vi "MultiplexDAQ_Main.vi"() -> ()   [LabVIEW 2011]
uses:
  controls/General Hardware config.ctl
  controls/DAQ Setup.ctl
  controls/PlotProperties.ctl
  controls/SampleClockExport.ctl
  controls/AnalogOutputSetup.ctl
  controls/RefClockSettings.ctl
  controls/Counter Setup.ctl
  controls/ProgramStatus.ctl
  <vilib>/Utility/miscctls.llb/LVBoundsTypeDef.ctl
  <vilib>/Utility/miscctls.llb/LVPointTypeDef.ctl
  <vilib>/Utility/miscctls.llb/LVRectTypeDef.ctl
  controls/XmlOption.ctl
  <vilib>/DAQmx/write.llb/DAQmx Write (Analog 1D DBL NChan 1Samp).vi
  <vilib>/DAQmx/read.llb/DAQmx Read (Analog 2D DBL NChan NSamp).vi
  <vilib>/DAQmx/miscellaneous.llb/DAQmx Fill In Error Info.vi
  C:/Program Files/National Instruments/LabVIEW 2011/resource/objmgr/daqmx.rc
panel:
  out "XMLConfigControls":refnum<vi>[](array[refnum])
  out "DisableDuringRecord":refnum<vi>[](array[refnum])
  in  "TDMS Group Name":string="MultiplexRecord"
  out "BufferStatus":u32[](array[colorbox])
  out "DisableDuringRun":refnum<vi>[](array[refnum])
  out "AllTasks":T1
  out "KillEvent":refnum<user-event>[](array[refnum])
  in  "Tab Control":T2(tab)=enum."Raw Signal"
  in  "Note":string
  out "Recording Time":string
  out "Index":i32
  in  "Menu Ring":enum16{"Manual", "Column"}(ring)
  in  "Up Button":bool
  in  "Down Button":bool
  in  "Preview?":bool
  in  "OverWrite?":bool
  in  "StartRecord":bool
  out "Amplitude Scale":dbl
  out "Effective Sampling Rate":dbl
  in  "Plot Properties":T3={"First Index"=0, "Last Index"=10, "Time (sec)"=1.0, "Zoom Factor"=1.0, "SubtractMean?"=FALSE, "DisplayOption"=enum."Scroll"} {"Zoom Factor" min=0.0 max=1.0}
  in  "TDMS file path":path=path "C:/Users/DAQ/Desktop/test_001.tdms"
  out "Waveform Graph":dbl[][](graph)
  in  "AutoNr":bool
  in  "SingleRaw?":bool
  in  "AC/DC Select":T4(ring)
  in  "WindowSize":i32=1 caption="(s)  Window Size For Averaging" min=1 max=10
  out "Intensity Graph":dbl[][](graph) caption="Array"
  in  "Row/Col Index":dbl caption="Select the Row/Col Index" min=0.0
  in  "Row/Col Select":enum16{"Show single column", "Show single row"}(ring)
  out "DC Offset":dbl[](graph) caption="Mean of Signal during window"
  out "AC_Range":dbl[](graph) caption="Standard Deviation of Signal during window"
  out "Raw Signal":dbl[](graph)
  in  "Raw Channel":i32=6 caption="Select Column" min=0
  in  "Open Button":bool
  in  "Save Button":bool
  in  "LUT":i32[](array[numeric]) caption="Channel Mix Vector"
  in  "BitSwitch":bool=TRUE caption="Switch most/least Significant bit"
  in  "HWSettings":T5={"Nr. of Columns"=1, "Nr. of Rows"=18, "OverSampling"=10, "Fetch Rate "=20, "Sampling Rate"=50000, "Nr. of BNC inputs"=3, "Sample Strip Length"=1} caption="Hardware Settingss"
  out "Smpls per Poll":i32 caption="Effective samples \nper poll"
  out "Smpls per CH*poll":i32 caption="Smpls per channel \nper poll"
  in  "AnalogSettings":T6=[{"AnalogOut (Volt)"=[5.0, 5.0, 5.0, 5.0], "DAQmx Device Name"="PXI1Slot2"}, {"AnalogOut (Volt)"=[5.0, 5.0, 5.0, 5.0], "DAQmx Device Name"="PXI1Slot3"}, {"AnalogOut (Volt)"=[5.0, 5.0, 5.0, 5.0], "DAQmx Device Name"="PXI1Slot6"}] caption="Analog Output Voltage Setup"
  in  "Digital Out Tasks":tag[](array[tag])=["PXI1Slot2/port0", "PXI1Slot3/port0", "PXI1Slot6/port0"]
  in  "Referece Clock Setup":T7={"RefClockGlobalName"="PXI_Clk10", "RefClockRate"=10000000.0}
  in  "Counter Setup":T8={"Device and Counter"="PXI1Slot3/ctr0", "PXI_trigger"="PXI_Trig3"}
  in  "RowConfigFile":path=path "C:/Users/DAQ/Desktop/Labview Joost/MultiplexDAQ/ConfigFiles/DecBinVals_L2R.txt" caption="Row Select Configuration file"
  in  "AnalogInSettings":T9[](array[typedef])=[{"Input Voltage Range"=10.0, "Upsample Coefficient"=1, "Analog Input Channels"="PXI1Slot2/ai0:7", "Configuration"=10106}, {"Input Voltage Range"=10.0, "Upsample Coefficient"=1, "Analog Input Channels"="PXI1Slot3/ai0:7", "Configuration"=10106}, {"Input Voltage Range"=10.0, "Upsample Coefficient"=2, "Analog Input Channels"="PXI1Slot6/ai0:4", "Configuration"=10106}] caption="Analog Input Tasks per PXI device" {"Configuration" items=["Differential"=10106, "RSE"=10083, "NRSE"=10078, "Pseudodifferential"=12529]}
  out "Digital Out BitMask":bool[][][](array[boolean])
  in  "Sample Clock Export":T10={"DAQmx Terminal"="/PXI1Slot2/PFI0", "ExportClock?"=FALSE, "DAQmx Device Name"="PXI1Slot2"}
  # "Plot Window Settings"
  # "V/unit"
  # "Hz"
  # "Disclaimer:\nThe mean and standard deviation\nthat are displayed in the graphs are\nan approximation of the real mean\nand standard deviation. \n\nUse Matlab to calculate the real values\nif they are important."
  # "Analog Input Settings"
  # "Analog Output Settings"
  # "General Hardware Settings"
  # "Row Select Digital Output Setting"
  # "Array"
  # "Acq. System"
  # "Other analog Input"
  # "You can export the sampling clock of any task to a DAQmx terminal. This is usefull for testing with the scope."
  # "Select PXI card"
  # "Time"
  # "Bit"
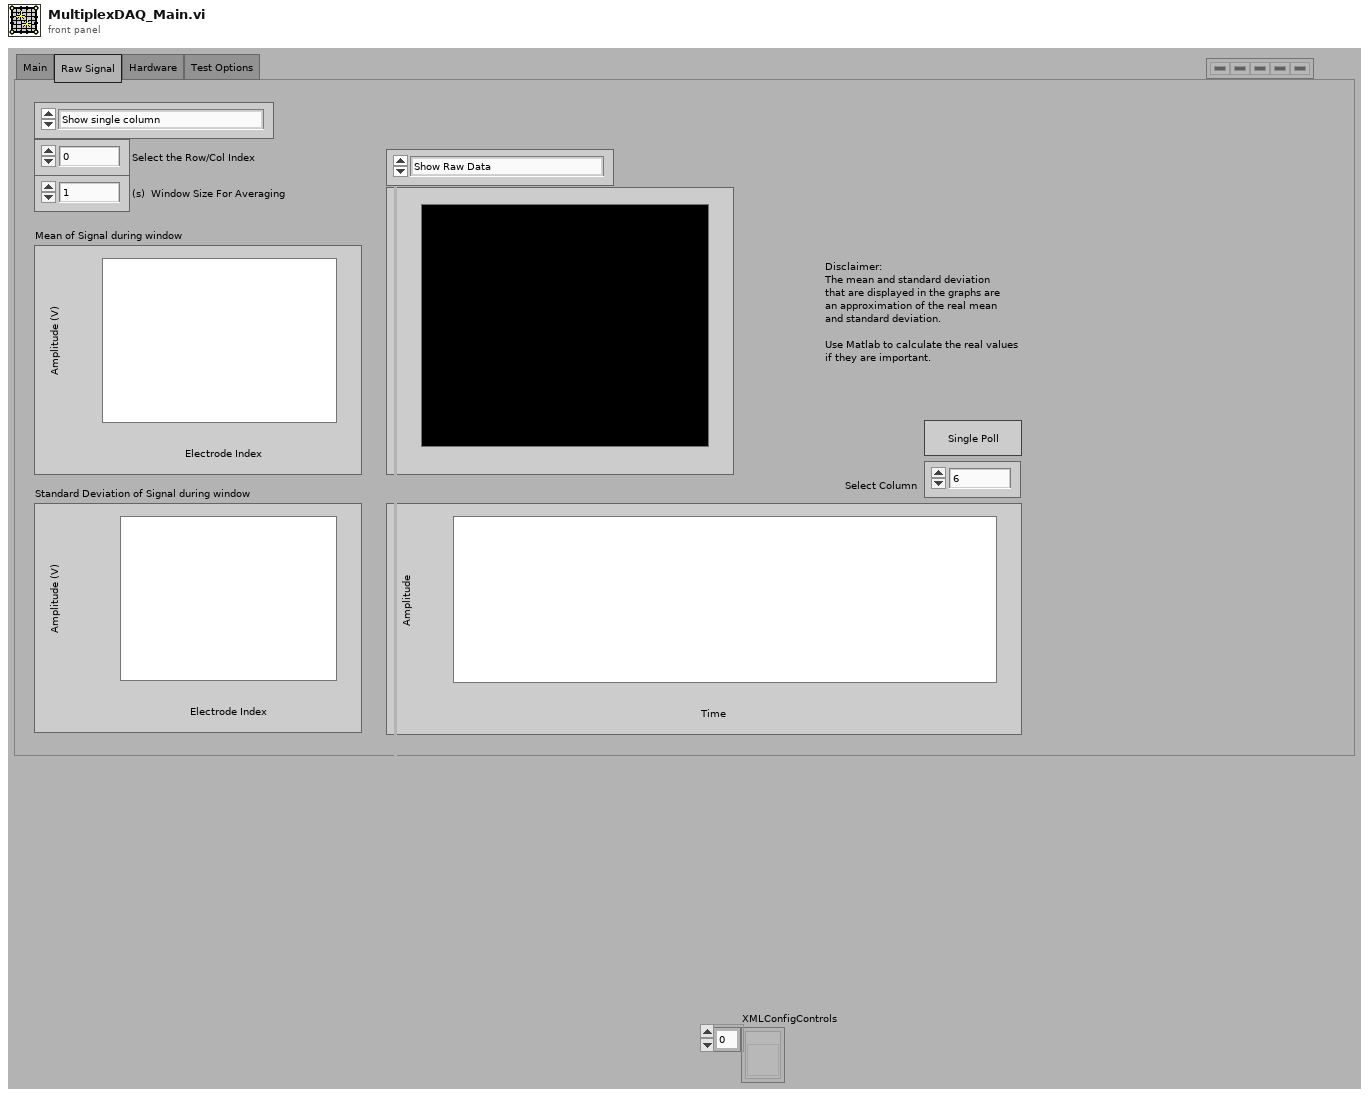
[diagram p1: front panel]
types:
  T1 = cluster{"tdms file out":refnum<k34>, "Tasks Out":refnum<k21>[], "DigitalTasks OUT":refnum<k21>[], "AnalogTaskOut":refnum<k21>[], "StartCounter":u32}
  T2 = enum32{"Main", "Raw Signal", "Hardware", "Test Options"}
  T3 = typedef "PlotProperties.ctl" = cluster{"First Index":i32, "Last Index":i32, "Time (sec)":dbl, "Zoom Factor":dbl, "SubtractMean?":bool, "DisplayOption":enum16{"Scroll", "Monitor"}}
  T4 = enum16{"Show Raw Data", "Show DC Offset", "Show AC Range"}
  T5 = typedef "General Hardware config.ctl" = cluster{"Nr. of Columns":i32, "Nr. of Rows":i32, "OverSampling":i32, "Fetch Rate ":i32, "Sampling Rate":i32, "Nr. of BNC inputs":i32, "Sample Strip Length":i32}
  T6 = typedef "AnalogOutputSetup.ctl" = cluster{"AnalogOut (Volt)":dbl[], "DAQmx Device Name":tag}[]
  T7 = typedef "RefClockSettings.ctl" = cluster{"RefClockGlobalName":string, "RefClockRate":dbl}
  T8 = typedef "Counter Setup.ctl" = cluster{"Device and Counter":tag, "PXI_trigger":string}
  T9 = typedef "DAQ Setup.ctl" = cluster{"Input Voltage Range":dbl, "Upsample Coefficient":u32, "Analog Input Channels":tag, "Configuration":i32}
  T10 = typedef "SampleClockExport.ctl" = cluster{"DAQmx Terminal":tag, "ExportClock?":bool, "DAQmx Device Name":tag}
  T11 = typedef "ProgramStatus.ctl" = enum16{"Init", "Init2", "Run", "Close"}
  T12 = cluster{"tdms file out":refnum<k34>, "Tasks Out":refnum<k21>[], "DigitalTasks OUT":refnum<k21>[], "AnalogOut":refnum<k21>[]}
  T13 = cluster{"tdms file out":refnum<k34>, "Tasks Out":refnum<k21>[], "DigitalTasks OUT":refnum<k21>[], "AnalogOut":refnum<k21>[], dbl}
  T14 = cluster{"Upsample Coefficient":u32, "NrChannels":i32, "First Channel Index":i32}
  T15 = enum8{"Enabled", "Disabled", "Disabled and Grayed Out"}
  T16 = typedef "LVBoundsTypeDef.ctl" = cluster{"Width":u32, "Height":u32}
  T17 = typedef "LVPointTypeDef.ctl" = cluster{"Horizontal":i16, "Vertical":i16}
  T18 = enum16{"open", "open or create", "create or replace", "create", "open (read-only)"}
  T19 = typedef "XmlOption.ctl" = enum16{"Save Custom", "Load Custom", "Save Default", "Load Default"}
  T20 = typedef "LVRectTypeDef.ctl" = cluster{"Left":i16, "Top":i16, "Right":i16, "Bottom":i16}
  T21 = cluster{"left":bool, "top":bool, "right":bool, "bottom":bool}
  T22 = typedef "LVPositionTypeDef.ctl" = cluster{"Left":i32, "Top":i32}
  T23 = cluster{"tdms file out":refnum<k34>, "Tasks Out":refnum<k21>[], "DigitalTasks OUT":refnum<k21>[], "AnalogTaskOut":refnum<k21>[]}
  T24 = cluster{"tdms file out":refnum<k34>, "Tasks Out":refnum<k21>[], "DigitalTasks OUT":refnum<k21>[], "AnalogTaskOut":refnum<k21>[], dbl}
  T25 = cluster{"First Index":i32, "Last Index":i32, "Time (sec)":dbl, "Zoom Factor":dbl, "SubtractMean?":bool, "DisplayOption":enum16{"Scroll", "Monitor"}}
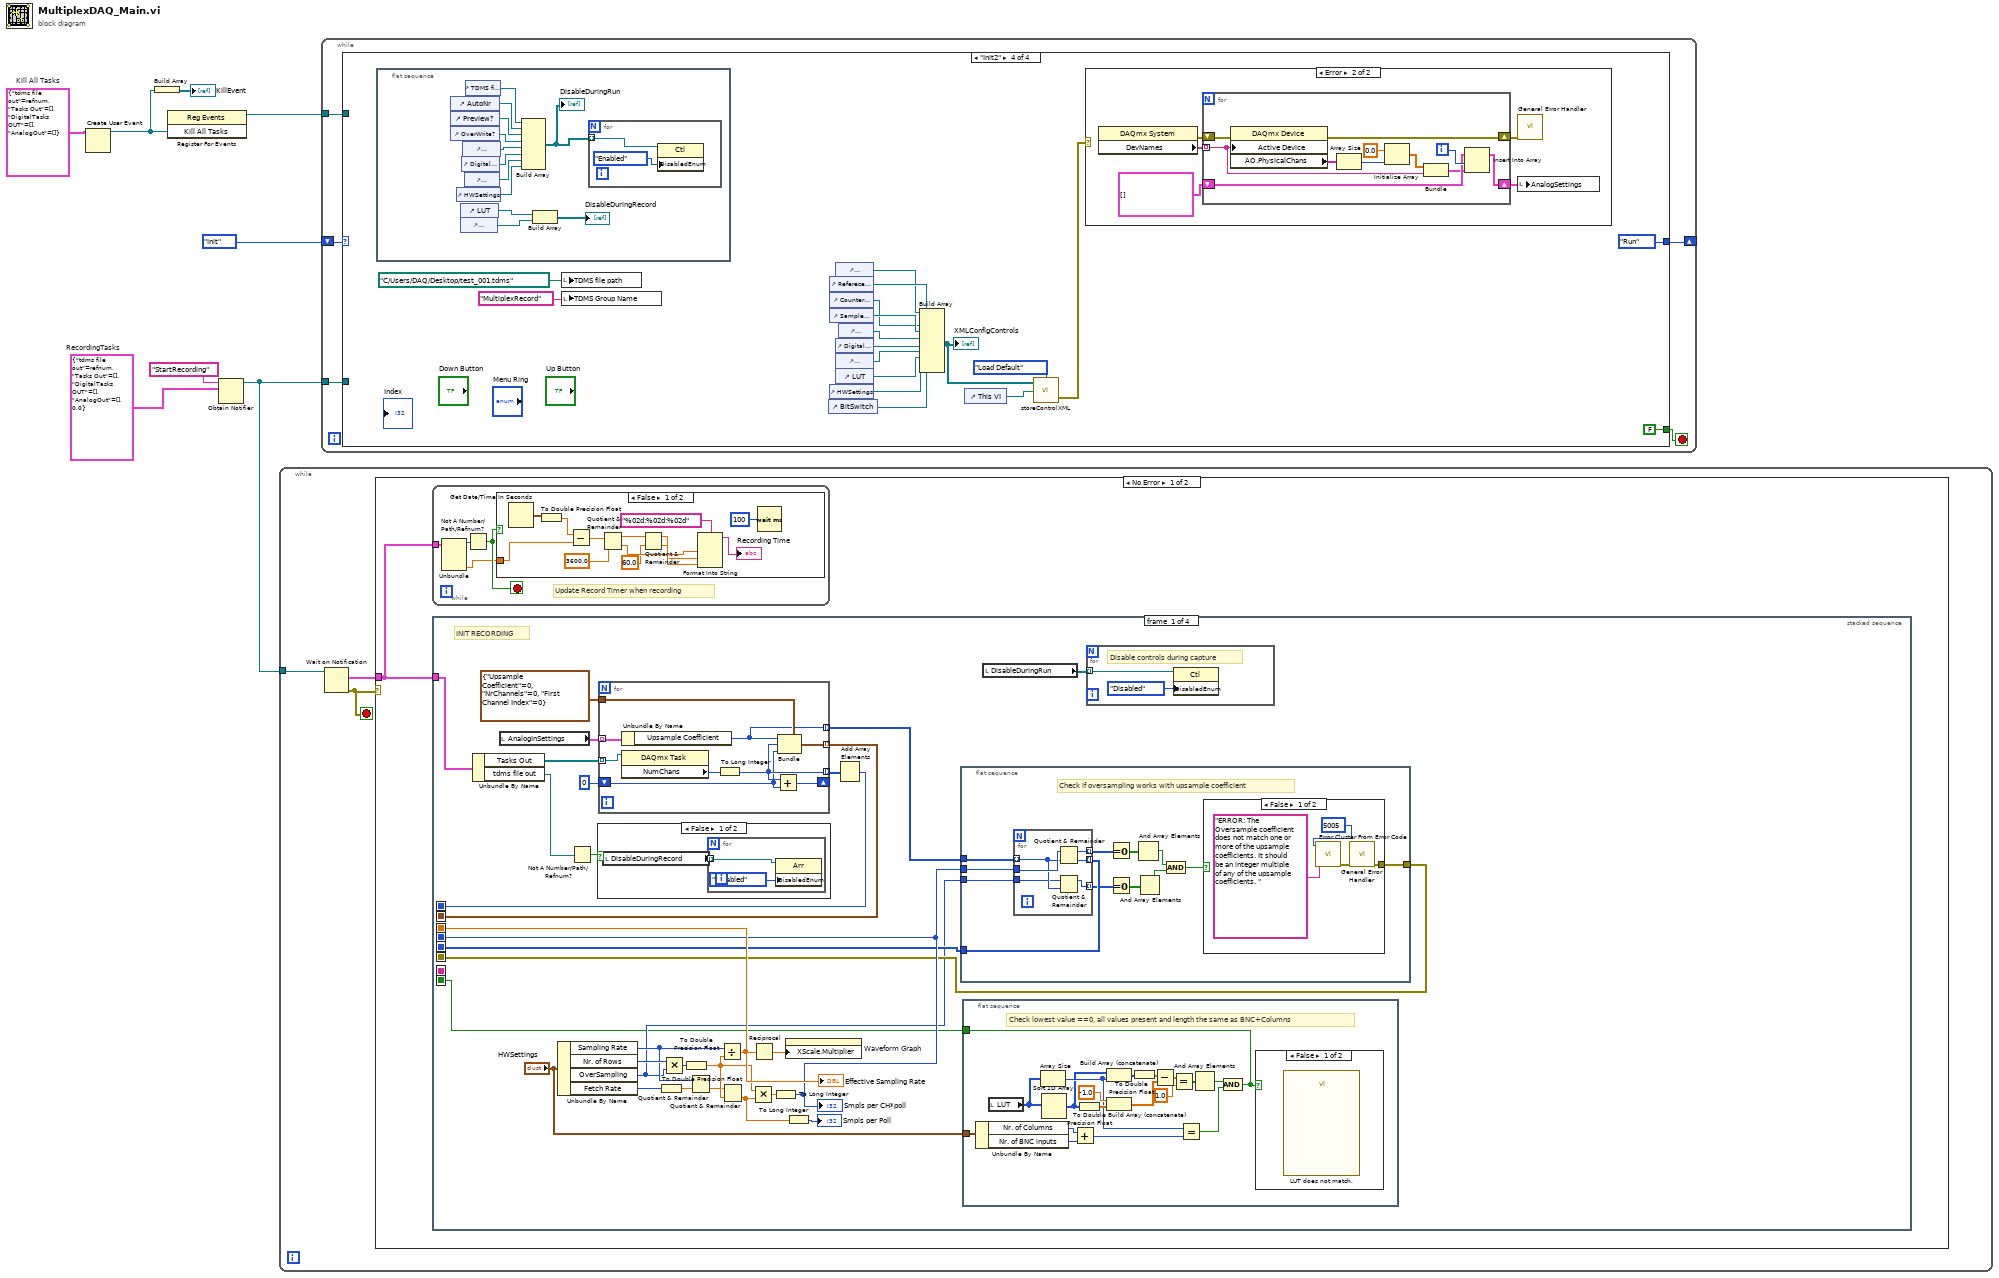
[diagram p0: block diagram]
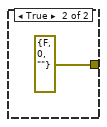
[diagram p4: hidden frame]
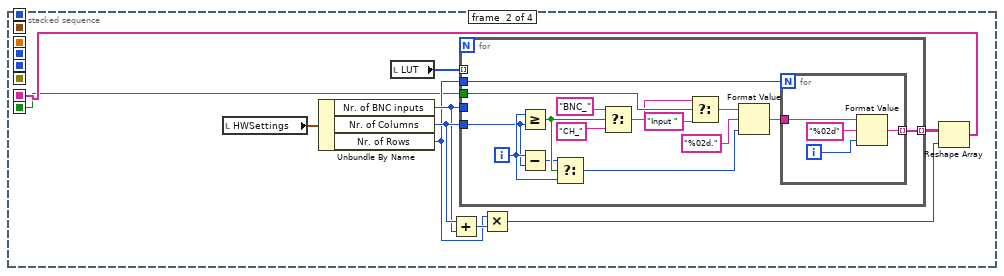
[diagram p6: hidden frame]
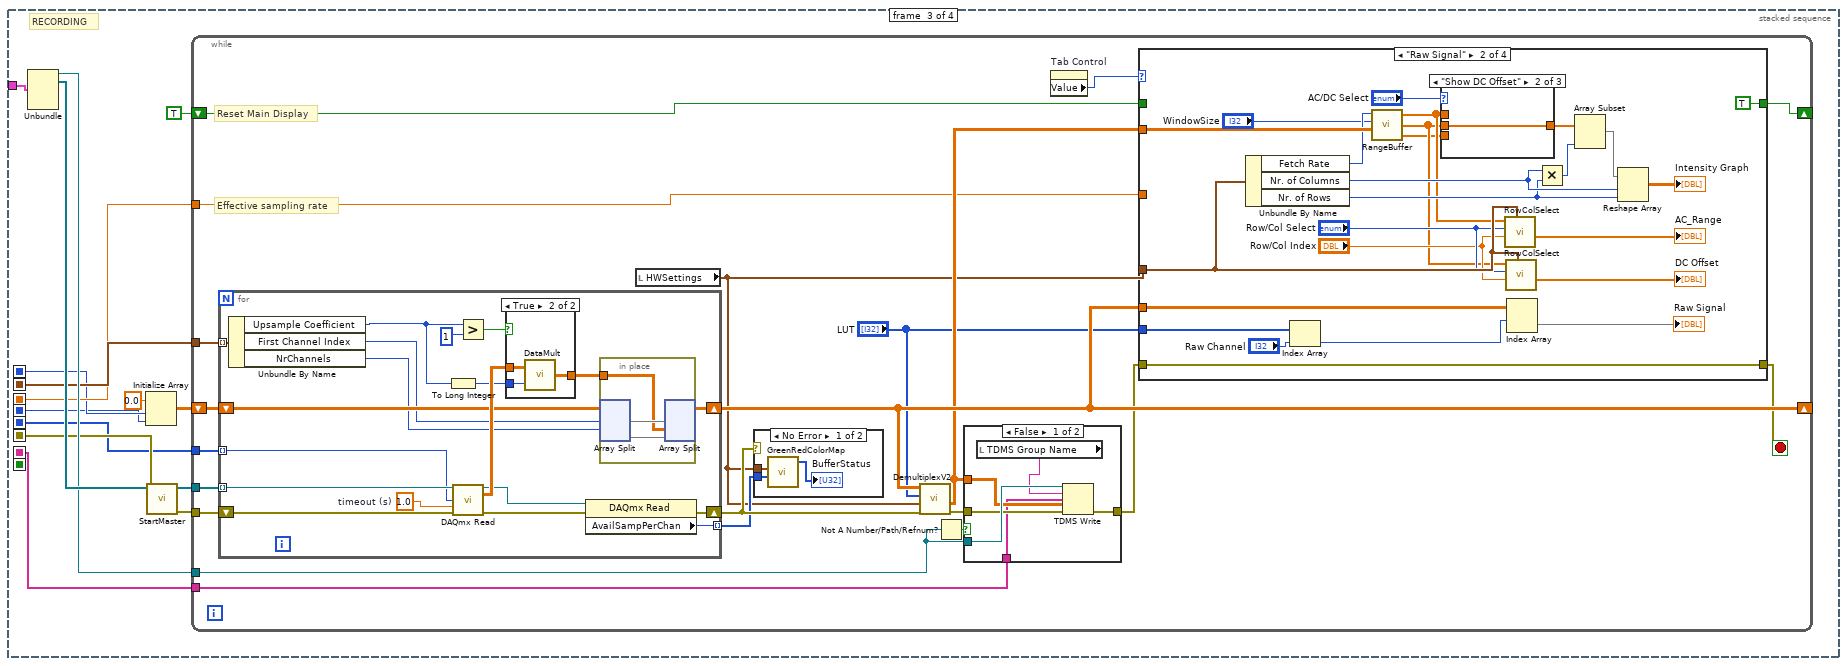
[diagram p7: hidden frame]
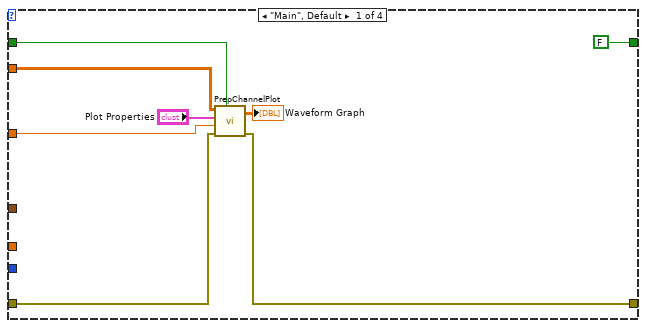
[diagram p9: hidden frame]
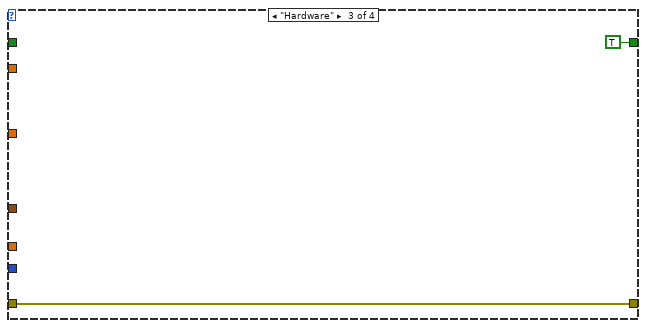
[diagram p12: hidden frame]
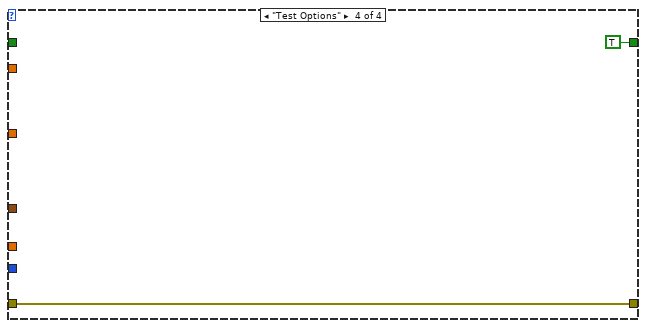
[diagram p13: hidden frame]
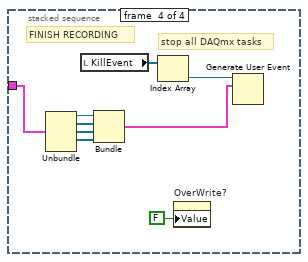
[diagram p16: hidden frame]
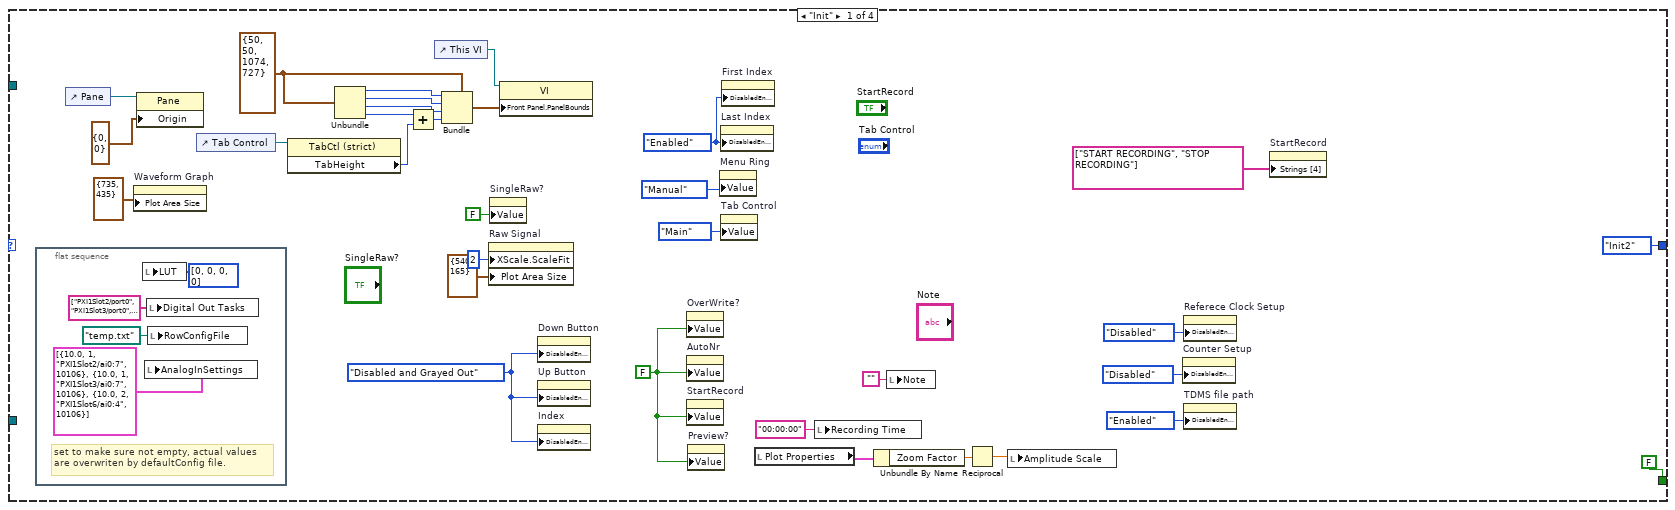
[diagram p18: hidden frame]
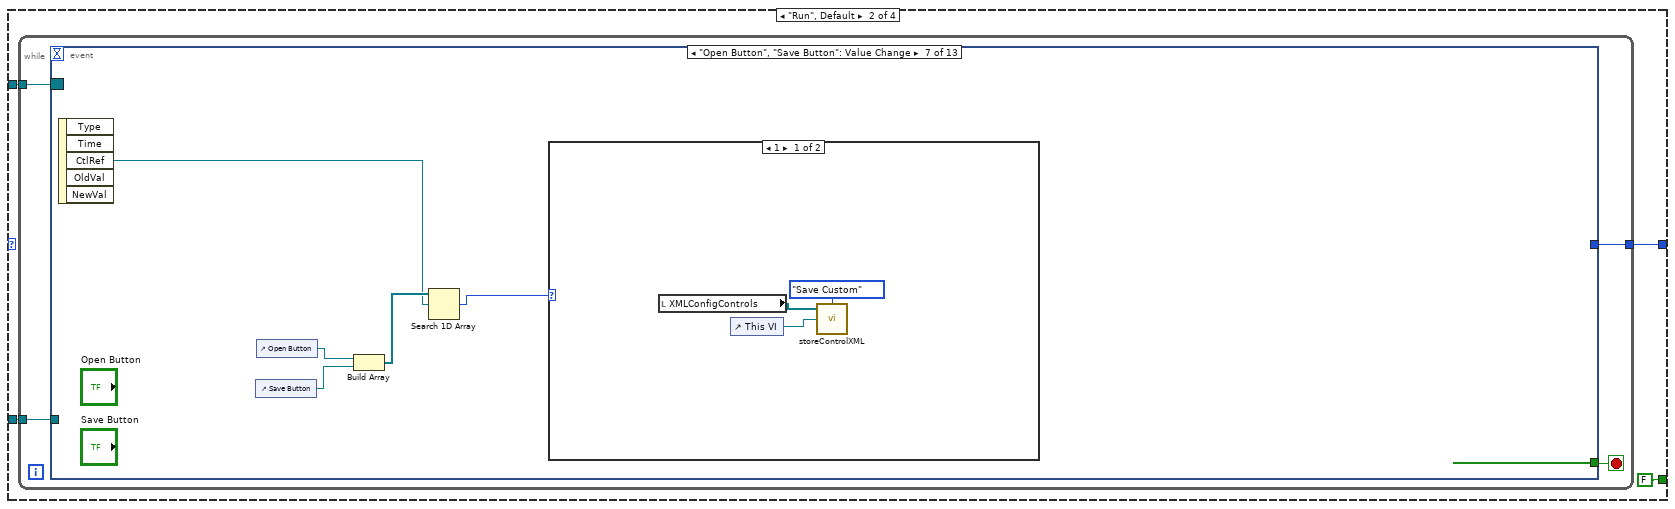
[diagram p19: hidden frame]
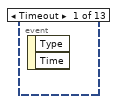
[diagram p20: hidden frame]
diagram:
  w1 = T12 {"tdms file out"=refnum, "Tasks Out"=[], "DigitalTasks OUT"=[], "AnalogOut"=[]}  # Kill All Tasks
  w6 = T13 {"tdms file out"=refnum, "Tasks Out"=[], "DigitalTasks OUT"=[], "AnalogOut"=[], 0.0}  # RecordingTasks
  n1 = Create User Event(user event datatype=w1) -> (user event=w4:refnum<user-event>)  [unwired: 1 in, 1 out]
  n2 = Build Array(w4) -> (→"KillEvent":refnum<user-event>[])
  n3 = register-events(w4) -> (reference out=w5:refnum<event-registration>)  [unwired: 2 in, 1 out]
  n4 = Obtain Notifier(name (unnamed)="StartRecording", notification data type=w6) -> (notifier out=w7:refnum<notifier>)  [unwired: 2 in, 2 out]
  n5 = while {
    tunnel: w7 -> [w9]
    stop <- w10 stop-if-true
    n6 = Wait on Notification(notifier=w9) -> (notification=w11:T13, error out=w10:errorcluster)  [unwired: 3 in, 2 out]
    n7 = case shown="No Error" w10 {
      tunnel: w11 -> [w12 _]
      frame No Error {
        n8 = while {
          tunnel: w12 -> [w16]
          stop <- w14 stop-if-true
          # "Update Record Timer when recording"
          n9 = Unbundle(w16) -> ("tdms file out"=w15:refnum<k34>, w13:dbl)  [unwired: 3 out]
          n10 = Not A Number/Path/Refnum?(number/path/refnum=w15) -> (NaN/Path/Refnum?=w14:bool)
          n11 = case shown="False" w14 {
            tunnel: w13 -> [w26 _]
            frame False {
              n12 = Get Date/Time In Seconds() -> (seconds since 1Jan1904=w28:timestamp)
              n13 = To Double Precision Float(number=w28) -> (double precision float=w27:dbl)
              n14 = Subtract(x=w27, y=w26) -> (x-y=w25:dbl)
              n15 = Quotient & Remainder(x=w25, y=3600.0) -> (x-y*floor(x/y)=w24:dbl, floor(x/y)=w20:dbl)
              n16 = Quotient & Remainder(x=w24, y=60.0) -> (x-y*floor(x/y)=w22:dbl, floor(x/y)=w21:dbl)
              n17 = Format Into String(format string="%02d:%02d:%02d", w20, w21, w22) -> (resulting string=→"Recording Time":string)  [unwired: 2 in, 1 out]
              n18 = Wait (ms)(milliseconds to wait=u32 100) -> ()  [unwired: 1 out]
            }
            frame True {
            }
          }
        }
        n19 = stacked-sequence {
          seq-local: [w50 _ _ _] -> [_ _ w150 _]
          seq-local: [w52 _ _ _] -> [_ _ w151 _]
          seq-local: [w36 _ _ _] -> [_ _ w149 _]
          seq-local: [w51 _ _ _] -> [_ _ w152 _]
          seq-local: [w35 _ _ _] -> [_ _ w146 _]
          seq-local: [w34 _ _ _] -> [_ _ w145 _]
          seq-local: [_ w116 _ _] -> [_ _ w144 _]
          seq-local: [w32 _ _ _] -> [_ w115 _ _]
          tunnel: w12 -> [w47 _ w157 w262]
          frame #0 {
            # "INIT RECORDING"
            n20 = Unbundle By Name(w47) -> ("Tasks Out"=w46:refnum<k21>[], "tdms file out"=w30:refnum<k34>)
            n21 = local read "AnalogInSettings"() -> (w48:T9[])
            n22 = Unbundle By Name("HWSettings") -> ("Sampling Rate"=w45:i32, "Nr. of Rows"=w56:i32, "OverSampling"=w33:i32, "Fetch Rate"=w57:i32)
            n23 = Not A Number/Path/Refnum?(number/path/refnum=w30) -> (NaN/Path/Refnum?=w31:bool)
            n24 = case shown="False" w31 {
              frame False {
                n25 = local read "DisableDuringRecord"() -> (w60:refnum<vi>[])
                n26 = for {
                  tunnel: w60 -> [w62] mode=indexing
                  n27 = property class="Arr"(reference=w62, "DisabledEnum"=T15."Disabled" ("Disabled")) -> ()  [unwired: 1 in, 2 out]
                }
              }
              frame True {
              }
            }
            n28 = for {
              tunnel: w46 -> [w112] mode=indexing
              tunnel: [w109] -> w53 mode=indexing
              shift-right: [w107] -> _
              shift-left: 0 -> [w108]
              tunnel: w48 -> [w113] mode=indexing
              tunnel: [w111] -> w51 mode=indexing
              tunnel: T14 {"Upsample Coefficient"=0, "NrChannels"=0, "First Channel Index"=0} ("cluster") -> [w110]
              tunnel: [w106] -> w37 mode=indexing
              n29 = property class="DAQmx Task"(reference=w112) -> ("NumChans"=w114:u32)  [unwired: 1 in, 2 out]
              n30 = Unbundle By Name(w113) -> ("Upsample Coefficient"=w106:u32)
              n31 = To Long Integer(number=w114) -> (32bit integer=w109:i32)
              n32 = Add(x=w109, y=w108) -> (x+y=w107:i32)
              n33 = Bundle(cluster=w110, "Upsample Coefficient"=w106, "NrChannels"=w109, "First Channel Index"=w108) -> (w111:T14)
            }
            n34 = To Double Precision Float(number=w57) -> (double precision float=w42:dbl)
            n35 = Multiply(x=w56, y=w33) -> (x*y=w58:i32)
            n36 = To Double Precision Float(number=w58) -> (double precision float=w40:dbl)
            n37 = Quotient & Remainder(x=w45, y=w42) -> (floor(x/y)=w38:dbl)  [unwired: 1 out]
            n38 = Divide(x=w45, y=w40) -> (x/y=w52:dbl)
            "Effective Sampling Rate" <- w52
            n39 = Quotient & Remainder(x=w38, y=w40) -> (floor(x/y)=w41:dbl)  [unwired: 1 out]
            n40 = Multiply(x=w40, y=w41) -> (x*y=w49:dbl)
            n41 = Reciprocal(x=w52) -> (1/x=w59:dbl)
            n42 = To Long Integer(number=w49) -> (32bit integer=w36:i32)
            "Smpls per CH*poll" <- w36
            n43 = property on="Waveform Graph" class="WFGraph (strict)"("XScale.Multiplier"=w59) -> ()  [unwired: 2 in, 2 out]
            n44 = To Long Integer(number=w41) -> (32bit integer=→"Smpls per Poll":i32)
            n45 = Add Array Elements(numeric array=w53) -> (sum=w50:i32)
            n46 = flat-sequence {
              tunnel: w37 -> [w74]
              tunnel: w36 -> [w73]
              tunnel: [w71] -> w35
              tunnel: [w70] -> w34
              tunnel: w33 -> [w69]
              frame #0 {
                # "Check if oversampling works with upsample coefficient"
                n47 = for {
                  tunnel: w74 -> [w83] mode=indexing
                  tunnel: w73 -> [w85]
                  tunnel: [w84] -> w70 mode=indexing
                  tunnel: w69 -> [w82]
                  tunnel: [w81] -> w68 mode=indexing
                  tunnel: [w80] -> w67 mode=indexing
                  n48 = Quotient & Remainder(x=w85, y=w83) -> (x-y*floor(x/y)=w80:u32, floor(x/y)=w84:u32)
                  n49 = Quotient & Remainder(x=w82, y=w83) -> (x-y*floor(x/y)=w81:u32)  [unwired: 1 out]
                }
                n50 = Equal To 0?(x=w67) -> (x = 0?=w66:bool[])
                n51 = Equal To 0?(x=w68) -> (x = 0?=w72:bool[])
                n52 = And Array Elements(Boolean array=w66) -> (logical AND=w65:bool)
                n53 = And Array Elements(Boolean array=w72) -> (logical AND=w64:bool)
                n54 = And(x=w65, y=w64) -> (x .and. y?=w63:bool)
                n55 = case shown="False" w63 {
                  tunnel: [w75 errorcluster {"status"=FALSE, "code"=0, "source"=""} ("error out")] -> w71
                  frame False {
                    n56 = call <vilib>:"Error Cluster From Error Code.vi"("error message (\"\")"="ERROR: The Oversample coefficient does not match one or more of the upsample coefficients. It should be an integer multiple of any of the upsample coefficients. " ("error message (\"\")"), "error code (0)"=5005) -> ("error out"=w76:errorcluster)  [unwired: 7 in]
                    n57 = call <vilib>:"General Error Handler.vi"("error in (no error)"=w76) -> ("error out"=w75:errorcluster)  [unwired: 10 in, 4 out]
                  }
                  frame True {
                  }
                }
              }
            }
            n58 = flat-sequence {
              tunnel: "HWSettings" -> [w103]
              tunnel: [w91] -> w32
              frame #0 {
                # "Check lowest value ==0, all values present and length the same as BNC+Columns"
                n59 = Unbundle By Name(w103) -> ("Nr. of Columns"=w101:i32, "Nr. of BNC inputs"=w102:i32)
                n60 = local read "LUT"() -> (w99:i32[])
                n61 = Array Size(array=w99) -> (size(s)=w89:i32)
                n62 = Sort 1D Array(array=w99) -> (sorted array=w87:i32[])
                n63 = Add(x=w101, y=w102) -> (x+y=w94:i32)
                n64 = To Double Precision Float(number=w87) -> (double precision float=w92:dbl[])
                n65 = Build Array (concatenate)(w87, w89) -> (w90:i32[])
                n66 = Build Array (concatenate)(-1.0, w92) -> (w98:dbl[])
                n67 = To Double Precision Float(number=w90) -> (double precision float=w86:dbl[])
                n68 = Subtract(x=w86, y=w98) -> (x-y=w97:dbl[])
                n69 = Equal?(x=w97, y=1.0) -> (x = y?=w95:bool[])
                n70 = Equal?(x=w89, y=w94) -> (x = y?=w93:bool)
                n71 = And Array Elements(Boolean array=w95) -> (logical AND=w88:bool)
                n72 = Compound Arithmetic op=AND(w88, w93) -> (w91:bool)
                n73 = case shown="False" w91 {
                  frame False {
                    n74 = call "LUT does not match."() -> ()  [unwired: 10 in, 2 out]
                  }
                  frame True {
                  }
                }
              }
            }
            n75 = local read "DisableDuringRun"() -> (w44:refnum<vi>[])
            n76 = for {
              tunnel: w44 -> [w105] mode=indexing
              # "Disable controls during capture"
              n77 = property class="Ctl"(reference=w105, "DisabledEnum"=T15."Disabled" ("Disabled")) -> ()  [unwired: 1 in, 2 out]
            }
          }
          frame #1 {
            n78 = local read "HWSettings"() -> (w124:T5)
            n79 = Unbundle By Name(w124) -> ("Nr. of BNC inputs"=w120:i32, "Nr. of Columns"=w121:i32, "Nr. of Rows"=w118:i32)
            n80 = local read "LUT"() -> (w123:i32[])
            n81 = Add(x=w121, y=w120) -> (x+y=w119:i32)
            n82 = for {
              tunnel: w123 -> [_] mode=indexing
              tunnel: w120 -> [_]
              tunnel: w121 -> [w134]
              tunnel: w118 -> [w130]
              tunnel: [w129] -> w122 mode=indexing
              tunnel: w115 -> [w128]
              i -> [w135]
              n83 = Greater Or Equal?(x=w135, y=w134) -> (x >= y?=w136:bool)
              n84 = Subtract(x=w135, y=w134) -> (x-y=w133:i32)
              n85 = Select(t=w133, s=w136, f=w135) -> (s? t:f=w132:i32)
              n86 = Select(t="BNC_", s=w136, f="CH_") -> (s? t:f=w126:string)
              n87 = Select(t=w126, s=w128, f="Input " ("t")) -> (s? t:f=w127:string)
              n88 = Format Value(string ("")=w127, format string="%02d.", value (0)=w132) -> (output string=w131:string)
              n89 = for {
                N: w130 -> [_]
                tunnel: w131 -> [w141]
                tunnel: [w140] -> w129 mode=indexing
                i -> [w143]
                n90 = Format Value(string ("")=w141, format string="%02d", value (0)=w143) -> (output string=w140:string)
              }
            }
            n91 = Multiply(x=w118, y=w119) -> (x*y=w117:i32)
            n92 = Reshape Array(w122, w117) -> (w116:string[])
          }
          frame #2 {
            # "RECORDING"
            n93 = Unbundle(w157) -> ("tdms file out"=w155:refnum<k34>, "Tasks Out"=w156:refnum<k21>[])  [unwired: 3 out]
            n94 = Initialize Array(0.0 ("element"), w150, w149) -> (w154:dbl[][])
            n95 = call "StartMaster.vi"("error in (no error)"=w146, "Tasks In"=w156) -> ("error out"=w148:errorcluster, "Tasks Out"=w158:refnum<k21>[])  [unwired: 8 in]
            n96 = while {
              tunnel: w155 -> [w173]
              tunnel: w158 -> [w177]
              shift-right: [w171] -> _
              shift-left: w154 -> [w179]
              tunnel: w152 -> [w176]
              tunnel: w151 -> [w165]
              tunnel: w148 -> [w175]
              shift-right: [w166] -> _
              shift-left: TRUE -> [w167]
              tunnel: w145 -> [w164]
              tunnel: w144 -> [w163]
              stop <- w168 stop-if-true
              # "Effective sampling rate"
              # "Reset Main Display"
              n97 = for {
                shift-right: [w244] -> w171
                shift-left: w179 -> [w245]
                tunnel: w177 -> [w246] mode=indexing
                tunnel: [w242] -> w161 mode=indexing
                shift-right: [w235] -> w162
                shift-left: w175 -> [w239]
                tunnel: w176 -> [w238] mode=indexing
                tunnel: w164 -> [w230] mode=indexing
                w234 = 1.0  # timeout (s)
                n98 = Unbundle By Name(w238) -> ("Upsample Coefficient"=w237:u32, "First Channel Index"=w232:i32, "NrChannels"=w233:i32)
                n99 = To Long Integer(number=w237) -> (32bit integer=w231:i32)
                n100 = call-poly <vilib>:"DAQmx Read.vi"("task/channels in"=w246, "number of samples per channel"=w230, "timeout"=w234, "error in"=w239) -> ("task out"=w243:refnum<k21>, "data"=w247:dbl[][], "error out"=w236:errorcluster)  [unwired: 9 in]
                n101 = Greater?(x=w237, y=u32 1) -> (0:w240:bool)
                n102 = case shown="True" w240 {
                  tunnel: w247 -> [w252 w255]
                  tunnel: w231 -> [_ w254]
                  tunnel: [w252 w253] -> w241
                  frame False {
                  }
                  frame True {
                    n103 = call "DataMult.vi"("Divider"=w254, "Data IN"=w255) -> ("Data OUT"=w253:dbl[][])
                  }
                }
                n104 = property class="DAQmx Read"(reference=w243, error in=w236) -> (error out=w235:errorcluster, "AvailSampPerChan"=w242:u32)  [unwired: 1 out]
                n105 = in-place {
                  in-place-border: w241 -> [w250]
                  n106 = in-place-split #1(w245, w232, w233) -> (w251:dbl[][], w249:dbl[][])  [unwired: 1 out]
                  n107 = in-place-split #1(w251, w250, w249) -> (w244:dbl[][])  [unwired: 2 out]
                }
              }
              n108 = local read "HWSettings"() -> (w160:T5)
              n109 = case shown="No Error" w162 {
                tunnel: w161 -> [w181 _]
                tunnel: w160 -> [w180 _]
                frame No Error {
                  n110 = call "GreenRedColorMap.vi"("DATA IN"=w181, "HWSettings"=w180) -> ("ColorOut"=→"BufferStatus":u32[])  [unwired: 3 in, 1 out]
                }
                frame Error {
                }
              }
              n111 = call "DemultiplexV2.vi"("Error In"=w162, "General HardWare Constants"=w160, "Lookup Table"="LUT", "Data In"=w171) -> ("Error Out"=w178:errorcluster, "Data Out"=w170:dbl[][])  [unwired: 6 in]
              n112 = Not A Number/Path/Refnum?(number/path/refnum=w173) -> (NaN/Path/Refnum?=w174:bool)
              n113 = case shown="False" w174 {
                tunnel: w173 -> [w228 _]
                tunnel: w178 -> [w227 w229]
                tunnel: [w226 w229] -> w169
                tunnel: w170 -> [w225 _]
                tunnel: w163 -> [w224 _]
                frame False {
                  n114 = local read "TDMS Group Name"() -> (w223:string)
                  n115 = TDMS Write(0:w228, 5:w223, 7:w224, 9:w225, 11:w227) -> (15:w226:errorcluster)  [unwired: 1 in, 3 out]
                }
                frame True {
                }
              }
              n116 = property on="Tab Control" class="TabCtl (strict)"() -> ("Value"=w172:T2)  [unwired: 2 in, 2 out]
              n117 = case shown="\"Raw Signal\"" w172 {
                tunnel: w170 -> [w188 w215 _ _]
                tunnel: w160 -> [_ w213 _ _]
                tunnel: w171 -> [_ w202 _ _]
                tunnel: w169 -> [w187 w196 w219 w221]
                tunnel: [w186 w196 w219 w221] -> w168
                tunnel: w165 -> [w185 _ _ _]
                tunnel: w167 -> [w184 _ _ _]
                tunnel: [FALSE TRUE TRUE TRUE] -> w166
                tunnel: "LUT" -> [_ w193 _ _]
                frame "Main", Default {
                  n118 = call "PrepChannelPlot.vi"("Data In"=w188, "Plot Properties"="Plot Properties", "Effective Sampling Rate"=w185, "Error In"=w187, "Init"=w184) -> ("Data Out"=→"Waveform Graph":dbl[][], "Error Out"=w186:errorcluster)
                }
                frame "Raw Signal" {
                  n119 = Unbundle By Name(w213) -> ("Fetch Rate"=w214:i32, "Nr. of Columns"=w205:i32, "Nr. of Rows"=w204:i32)
                  n120 = Index Array(array=w193, index="Raw Channel") -> (element=w191:i32)
                  n121 = call "RangeBuffer.vi"("DATA Input"=w215, "WindowSize"="WindowSize", "Fetch Rate"=w214) -> ("Raw Data"=w198:dbl[], "Mean Average"=w199:dbl[], "Standard Deviation"=w200:dbl[])  [unwired: 1 in]
                  n122 = case shown="\"Show DC Offset\"" "AC/DC Select" {
                    tunnel: w200 -> [_ _ w218]
                    tunnel: w199 -> [_ w217 _]
                    tunnel: w198 -> [w216 _ _]
                    tunnel: [w216 w217 w218] -> w197
                    frame "Show Raw Data", Default {
                    }
                    frame "Show DC Offset" {
                    }
                    frame "Show AC Range" {
                    }
                  }
                  n123 = call "RowColSelect.vi"("HWSettings"=w213, "Row/Col Index"="Row/Col Index", "Row/Col Select"="Row/Col Select", "DATA IN"=w200) -> ("DATA OUT"=→"AC_Range":dbl[])  [unwired: 7 in]
                  n124 = call "RowColSelect.vi"("HWSettings"=w213, "Row/Col Index"="Row/Col Index", "Row/Col Select"="Row/Col Select", "DATA IN"=w199) -> ("DATA OUT"=→"DC Offset":dbl[])  [unwired: 7 in]
                  n125 = Index Array(array=w202, index (row)=w191) -> (element=→"Raw Signal":dbl[])  [unwired: 1 in]
                  n126 = Multiply(x=w205, y=w204) -> (x*y=w209:i32)
                  n127 = Array Subset(array=w197, length=w209) -> (w208:dbl[])  [unwired: 1 in]
                  n128 = Reshape Array(w208, w205, w204) -> (→"Intensity Graph":dbl[][])
                }
                frame "Hardware" {
                }
                frame "Test Options" {
                }
              }
            }
          }
          frame #3 {
            # "stop all DAQmx tasks"
            # "FINISH RECORDING"
            n129 = Unbundle(w262) -> ("tdms file out"=w261:refnum<k34>, "Tasks Out"=w260:refnum<k21>[], "DigitalTasks OUT"=w259:refnum<k21>[], "AnalogOut"=w258:refnum<k21>[])  [unwired: 1 out]
            n130 = local read "KillEvent"() -> (w264:refnum<user-event>[])
            n131 = Bundle("tdms file out"=w261, "Tasks Out"=w260, "DigitalTasks OUT"=w259, "AnalogOut"=w258) -> (w257:T12)  [unwired: 1 in]
            n132 = Index Array(array=w264) -> (element=w263:refnum<user-event>)  [unwired: 1 in]
            n133 = property on="OverWrite?" class="Bool (strict)"("Value"=FALSE ("OverWrite?")) -> ()  [unwired: 2 in, 2 out]
            n134 = Generate User Event(user event=w263, event data cluster=w257) -> ()  [unwired: 1 in, 2 out]
          }
        }
      }
      frame Error {
      }
    }
  }
  n135 = while {
    shift-right: [w265] -> _
    shift-left: ProgramStatus."Init" ("Program Stat") -> [w266]
    tunnel: w7 -> [w268]
    tunnel: w5 -> [w267]
    stop <- w269 stop-if-true
    n136 = case shown="\"Init2\"" w266 {
      tunnel: [FALSE FALSE TRUE FALSE] -> w269
      tunnel: w268 -> [_ w308 _ _]
      tunnel: w267 -> [_ w307 _ _]
      tunnel: [ProgramStatus."Init2" ("Program Stat") w306 ProgramStatus."Close" ("Program Stat") ProgramStatus."Run" ("Program Stat")] -> w265
      frame "Init" {
        w281 = T15."Disabled and Grayed Out" ("Disabled")
        w282 = T15."Enabled" ("Disabled")
        w288 = FALSE ("StartRecord")
        w299 = T20 {"Left"=50, "Top"=50, "Right"=1074, "Bottom"=727} ("Front Panel Window:Panel Bounds")
        n137 = flat-sequence {
          frame #0 {
            # "set to make sure not empty, actual values\nare overwriten by defaultConfig file."
            n138 = local write "LUT"(i32[] [0, 0, 0, 0] ("LUT")) -> ()
            n139 = local write "AnalogInSettings"(T9[] [{"Input Voltage Range"=10.0, "Upsample Coefficient"=1, "Analog Input Channels"="PXI1Slot2/ai0:7", "Configuration"=10106}, {"Input Voltage Range"=10.0, "Upsample Coefficient"=1, "Analog Input Channels"="PXI1Slot3/ai0:7", "Configuration"=10106}, {"Input Voltage Range"=10.0, "Upsample Coefficient"=2, "Analog Input Channels"="PXI1Slot6/ai0:4", "Configuration"=10106}] ("AnalogInSettings")) -> ()
            n140 = local write "Digital Out Tasks"(tag[] ["PXI1Slot2/port0", "PXI1Slot3/port0", "PXI1Slot6/port0"] ("Digital Out Tasks")) -> ()
            n141 = local write "RowConfigFile"(path "temp.txt" ("RowConfigFile")) -> ()
          }
        }
        n142 = control-ref of="Pane"() -> (w291:refnum<vi>)
        n143 = property on="Waveform Graph" class="WFGraph (strict)"("Plot Area Size"=T16 {"Width"=735, "Height"=435} ("Plot Area:Size")) -> ()  [unwired: 2 in, 2 out]
        n144 = property class="Pane"(reference=w291, "Origin"=T17 {"Horizontal"=0, "Vertical"=0}) -> ()  [unwired: 1 in, 2 out]
        n145 = control-ref of="Tab Control"() -> (w293:refnum<vi>)
        n146 = property class="TabCtl (strict)"(reference=w293) -> ("TabHeight"=w300:u32)  [unwired: 1 in, 2 out]
        n147 = Unbundle(w299) -> ("Left"=w298:i16, "Top"=w297:i16, "Right"=w296:i16, "Bottom"=w295:i16)
        n148 = Add(x=w295, y=w300) -> (x+y=w294:u32)
        n149 = control-ref of="This VI"() -> (w290:refnum<vi>)
        n150 = Bundle(cluster=w299, "Left"=w298, "Top"=w297, "Right"=w296, "Bottom"=w294) -> (w274:T20)
        n151 = property on="Raw Signal" class="WFGraph (strict)"("XScale.ScaleFit"=u8 2 ("X Scale.Scale Fit"), "Plot Area Size"=T16 {"Width"=540, "Height"=165} ("Plot Area:Size")) -> ()  [unwired: 2 in, 2 out]
        n152 = property on="SingleRaw?" class="Bool (strict)"("Value"=FALSE ("SingleRaw?")) -> ()  [unwired: 2 in, 2 out]
        n153 = property class="VI"(reference=w290, "Front Panel.PanelBounds"=w274) -> ()  [unwired: 1 in, 2 out]
        n154 = property on="Down Button" class="Bool (strict)"("DisabledEnum"=w281) -> ()  [unwired: 2 in, 2 out]
        n155 = property on="Up Button" class="Bool (strict)"("DisabledEnum"=w281) -> ()  [unwired: 2 in, 2 out]
        n156 = property on="Index" class="DigNum (strict)"("DisabledEnum"=w281) -> ()  [unwired: 2 in, 2 out]
        n157 = property on="OverWrite?" class="Bool (strict)"("Value"=w288) -> ()  [unwired: 2 in, 2 out]
        n158 = property on="AutoNr" class="Bool (strict)"("Value"=w288) -> ()  [unwired: 2 in, 2 out]
        n159 = property on="StartRecord" class="Bool (strict)"("Value"=w288) -> ()  [unwired: 2 in, 2 out]
        n160 = property on="Preview?" class="Bool (strict)"("Value"=w288) -> ()  [unwired: 2 in, 2 out]
        n161 = property on="Menu Ring" class="Enum (strict)"("Value"=enum16{"Manual", "Column"}."Manual" ("Menu Ring")) -> ()  [unwired: 2 in, 2 out]
        n162 = property on="Last Index" class="DigNum (strict)"("DisabledEnum"=w282) -> ()  [unwired: 2 in, 2 out]
        n163 = property on="Tab Control" class="TabCtl (strict)"("Value"=T2."Main" ("Tab Control")) -> ()  [unwired: 2 in, 2 out]
        n164 = property on="First Index" class="DigNum (strict)"("DisabledEnum"=w282) -> ()  [unwired: 2 in, 2 out]
        n165 = local read "Plot Properties"() -> (w285:T3)
        n166 = local write "Recording Time"("00:00:00" ("Recording Time")) -> ()
        n167 = Unbundle By Name(w285) -> ("Zoom Factor"=w284:dbl)
        n168 = local write "Note"("") -> ()
        n169 = Reciprocal(x=w284) -> (1/x=w283:dbl)
        n170 = local write "Amplitude Scale"(w283) -> ()
        n171 = property on="Counter Setup" class="Clust (strict)"("DisabledEnum"=T15."Disabled" ("Disabled")) -> ()  [unwired: 2 in, 2 out]
        n172 = property on="Referece Clock Setup" class="Clust (strict)"("DisabledEnum"=T15."Disabled" ("Disabled")) -> ()  [unwired: 2 in, 2 out]
        n173 = property on="TDMS file path" class="Path"("DisabledEnum"=T15."Enabled" ("Disabled")) -> ()  [unwired: 2 in, 2 out]
        n174 = property on="StartRecord" class="Bool (strict)"("Strings [4]"=string[] ["START RECORDING", "STOP RECORDING"]) -> ()  [unwired: 2 in, 2 out]
      }
      frame "Run", Default {
        n175 = while {
          tunnel: w308 -> [w312]
          tunnel: w307 -> [w311]
          tunnel: [w310] -> w306
          stop <- w313 stop-if-true
          n176 = event shown="[6] \"Open Button\", \"Save Button\": Value Change" {
            selector: w311 -> [_ _ _ _ _ _ _ _ _ _ _ _ _]
            dyn-events: _ -> [_ _ _ _ _ _ _ _ _ _ _ _ _]
            timeout: _ -> [_ _ _ _ _ _ _ _ _ _ _ _ _]
            tunnel: [_ w317 _ _ _ _ _ _ _ _ _ _ _] -> w313
            tunnel: w312 -> [_ w316 _ _ _ w369 _ _ _ _ _ _ _]
            tunnel: [_ w315 _ _ _ _ _ _ _ _ _ _ ProgramStatus."Run" ("Program Stat")] -> w310
            event Timeout {
              n177 = event-data() -> ()  [unwired: 1 in, 2 out]
            }
            event Panel Close? {
              n178 = event-data() -> ()  [unwired: 1 in, 3 out]
              n179 = local read "StartRecord"() -> (w318:bool)
              n180 = case shown="False" w318 {
                tunnel: [TRUE FALSE] -> w317
                tunnel: w316 -> [w321 _]
                tunnel: [ProgramStatus."Close" ("Program Stat") ProgramStatus."Run" ("Program Stat")] -> w315
                tunnel: [TRUE ("Discard?") TRUE ("Discard?")] -> w314
                frame False {
                  n181 = Release Notifier(notifier=w321) -> ()  [unwired: 2 in, 3 out]
                }
                frame True {
                  n182 = call "Display Message to User"() -> ()  [unwired: 10 in, 2 out]
                }
              }
              n183 = event-data("Discard?"=w314) -> ()  [unwired: 1 in, 1 out]
            }
            event Panel Resize {
              n184 = event-data() -> ("OldBnds"=w330:T20, "NewBnds"=w326:T20)  [unwired: 1 in, 5 out]
              n185 = Equal?(x=w326, y=w330) -> (x = y?=w329:T21)
              n186 = Cluster To Array(cluster=w329) -> (array=w328:bool[])
              n187 = And Array Elements(Boolean array=w328) -> (logical AND=w327:bool)
              n188 = case shown="True" w327 {
                tunnel: w326 -> [_ w357]
                frame False {
                }
                frame True {
                  n189 = property on="Raw Signal" class="WFGraph (strict)"() -> ("Position"=w333:T22)  [unwired: 2 in, 2 out]
                  n190 = Unbundle(w357) -> ("left"=w354:i16, "top"=w352:i16, "right"=w355:i16, "bottom"=w353:i16)
                  n191 = property on="Waveform Graph" class="WFGraph (strict)"() -> ("Position"=w356:T22)  [unwired: 2 in, 2 out]
                  n192 = Subtract(x=w355, y=w354) -> (x-y=w334:i16)
                  n193 = Subtract(x=w353, y=w352) -> (x-y=w335:i16)
                  n194 = Unbundle(w333) -> ("Left"=w331:i32, "Top"=w332:i32)
                  n195 = Unbundle(w356) -> ("Left"=w351:i32, "Top"=w350:i32)
                  n196 = Subtract(x=w335, y=w351) -> (x-y=w348:i32)
                  n197 = Subtract(x=w334, y=w350) -> (x-y=w347:i32)
                  n198 = Subtract(x=w334, y=w332) -> (x-y=w338:i32)
                  n199 = Subtract(x=w335, y=w331) -> (x-y=w337:i32)
                  n200 = Subtract(x=w348, y=45) -> (x-y=w346:i32)
                  n201 = Subtract(x=w347, y=95) -> (x-y=w345:i32)
                  n202 = Subtract(x=w338, y=30) -> (x-y=w340:i32)
                  n203 = Subtract(x=w337, y=160) -> (x-y=w339:i32)
                  n204 = Bundle(w345, w346) -> (w349:cluster{i32, i32})  [unwired: 1 in]
                  n205 = Bundle(w340, w339) -> (w336:cluster{i32, i32})  [unwired: 1 in]
                  n206 = property on="Waveform Graph" class="WFGraph (strict)"("Plot Area Size"=w349) -> ()  [unwired: 2 in, 2 out]
                  n207 = property on="Raw Signal" class="WFGraph (strict)"("Plot Area Size"=w336) -> ()  [unwired: 2 in, 2 out]
                }
              }
            }
            event "SingleRaw?": Value Change {
              n208 = event-data() -> ("NewVal"=w358:bool)  [unwired: 1 in, 4 out]
              n209 = case shown="True" w358 {
                frame False {
                  n210 = property on="Raw Signal" class="WFGraph (strict)"("XScale.ScaleFit"=u8 2 ("X Scale.Scale Fit")) -> ()  [unwired: 2 in, 2 out]
                }
                frame True {
                  n211 = local read "HWSettings"() -> (w363:T5)
                  n212 = Unbundle By Name(w363) -> ("Nr. of Rows"=w360:i32, "OverSampling"=w362:i32)
                  n213 = Multiply(x=w360, y=w362) -> (x*y=w361:i32)
                  n214 = property on="Raw Signal" class="WFGraph (strict)"("XScale.ScaleFit"=u8 0 ("X Scale.Scale Fit"), "XScale.Maximum"=w361, "XScale.Minimum"=0.0 ("X Scale.Range:Minimum")) -> ()  [unwired: 2 in, 2 out]
                }
              }
            }
            event Value Change {
              n215 = event-data() -> ("NewVal"=w366:dbl)  [unwired: 1 in, 4 out]
              n216 = Reciprocal(x=w366) -> (1/x=→"Amplitude Scale":dbl)
            }
            event "StartRecord": Value Change {
              n217 = event-data() -> ("CtlRef"=w368:refnum<vi>, "NewVal"=w370:bool)  [unwired: 1 in, 3 out]
              n218 = case shown="True" w370 {
                tunnel: w369 -> [_ w382]
                tunnel: w368 -> [_ w380]
                frame False {
                  n219 = local read "AllTasks"() -> (w372:T1)
                  n220 = local read "KillEvent"() -> (w378:refnum<user-event>[])
                  n221 = Unbundle(w372) -> ("tdms file out"=w373:refnum<k34>, "Tasks Out"=w374:refnum<k21>[], "DigitalTasks OUT"=w375:refnum<k21>[], "AnalogTaskOut"=w376:refnum<k21>[])  [unwired: 1 out]
                  n222 = Index Array(array=w378) -> (element=w377:refnum<user-event>)  [unwired: 1 in]
                  n223 = Bundle("tdms file out"=w373, "Tasks Out"=w374, "DigitalTasks OUT"=w375, "AnalogTaskOut"=w376) -> (w371:T23)  [unwired: 1 in]
                  n224 = Generate User Event(user event=w377, event data cluster=w371) -> ()  [unwired: 1 in, 2 out]
                }
                frame True {
                  # "In this case, the tasks will be initiated and the TDMS file will be opened.\nThe Tasks are terminated in the recording while loop after the TDMS \nreference is killed when the \"stop recording\" button is pressed."
                  # "Start Recording"
                  n225 = case shown="False" "Preview?" {
                    tunnel: [w391 _] -> w383
                    tunnel: [w390 refnum<k34> refnum ("tdms file out")] -> w381
                    frame False {
                      n226 = local read "TDMS Group Name"() -> (w385:string)
                      n227 = case shown="True" "AutoNr" {
                        tunnel: "TDMS file path" -> [w400 w402]
                        tunnel: [w400 w401] -> w397
                        frame False {
                        }
                        frame True {
                          n228 = call "AutoIncreasePath.vi"("TDMS file path"=w402) -> ("TDMS file path out"=w401:path)  [unwired: 3 in, 1 out]
                        }
                      }
                      n229 = Select(t=T18."create or replace" ("operation (0:open)"), s="OverWrite?", f=T18."create" ("operation (0:open)")) -> (s? t:f=w394:T18)
                      n230 = local read "AnalogInSettings"() -> (w386:T9[])
                      n231 = local read "AnalogSettings"() -> (w384:T6)
                      n232 = TDMS Open(10:w394, 11:w397) -> (0:w392:errorcluster, 3:w389:refnum<k34>)  [unwired: 4 in]
                      n233 = local write "TDMS file path"(w397) -> ()
                      n234 = local read "HWSettings"() -> (w388:T5)
                      n235 = local read "LUT"() -> (w387:i32[])
                      n236 = call "tdmsProperties.vi"("AnalogSettings"=w384, "TDMS Group Name"=w385, "AnalogInSettings"=w386, "HWSettings"=w388, "Error In"=w392, "LUT"=w387, "tdms file In"=w389) -> ("Error Out"=w391:errorcluster, "tdms file Out"=w390:refnum<k34>)  [unwired: 3 in]
                    }
                    frame True {
                      n237 = local write "Recording Time"("00:00:00" ("Recording Time")) -> ()
                      n238 = local write "Note"("") -> ()
                    }
                  }
                  n239 = case shown="No Error" w383 {
                    selector: w383 -> [_ w452]
                    tunnel: w382 -> [w429 _]
                    tunnel: w381 -> [w409 _]
                    tunnel: w380 -> [_ w453]
                    frame No Error {
                      n240 = local read "HWSettings"() -> (w421:T5)
                      n241 = call "ConfigStartCards.vi"("Sample Clock Export"="Sample Clock Export", "Reference Clock Properties"="Referece Clock Setup", "DAQ Setup Array"="AnalogInSettings", "General HardWare Constants"=w421) -> ("error out"=w427:errorcluster, "Tasks Out"=w431:refnum<k21>[])  [unwired: 1 in, 2 out]
                      n242 = call "initDigitalOutTasks.vi"("Digital Out - Config File"="RowConfigFile", "General HardWare Constants"=w421, "Digital Out Tasks"="Digital Out Tasks", "Reference Clock Properties"="Referece Clock Setup", "Error In"=w427, "Switch Bitorder?"="BitSwitch", "Counter Setup"="Counter Setup") -> ("Error Out"=w414:errorcluster, "BitMaskValues out"=w412:u32[][], "BitMask Out"=→"Digital Out BitMask":bool[][][], "DigitalTasks OUT"=w430:refnum<k21>[])  [unwired: 1 in]
                      n243 = Not A Number/Path/Refnum?(number/path/refnum=w409) -> (NaN/Path/Refnum?=w408:bool)
                      n244 = case shown="False" w408 {
                        tunnel: w414 -> [w437 w438]
                        tunnel: [w436 w438] -> w413
                        tunnel: w409 -> [w435 _]
                        tunnel: w412 -> [w434 _]
                        tunnel: "Digital Out Tasks" -> [w433 _]
                        tunnel: "TDMS Group Name" -> [w432 _]
                        frame False {
                          n245 = call "TDMSRowSelect.vi"("Digital Out Tasks"=w433, "Group Name"=w432, "Error In"=w437, "BitMaskValues in"=w434, "tdms file In"=w435) -> ("Error Out"=w436:errorcluster)  [unwired: 6 in]
                        }
                        frame True {
                        }
                      }
                      n246 = Get Date/Time In Seconds() -> (seconds since 1Jan1904=w407:timestamp)
                      n247 = call "SetAnalogOutput.vi"("Reference Clock Properties"="Referece Clock Setup", "Error In"=w413, "Analog Output Voltage Setup"="AnalogSettings") -> ("Error Out"=w416:errorcluster, "AnalogTaskOut"=w423:refnum<k21>[])  [unwired: 1 in]
                      n248 = To Double Precision Float(number=w407) -> (double precision float=w406:dbl)
                      n249 = Bundle("tdms file out"=w409, "Tasks Out"=w431, "DigitalTasks OUT"=w430, "AnalogTaskOut"=w423, w406) -> (w426:T24)  [unwired: 1 in]
                      "AllTasks" <- w426
                      n250 = call <vilib>:"General Error Handler.vi"("error in (no error)"=w416) -> ("error out"=w417:errorcluster)  [unwired: 10 in, 4 out]
                      n251 = case shown="No Error" w417 {
                        selector: w417 -> [_ w447]
                        tunnel: w429 -> [w440 _]
                        tunnel: w426 -> [w439 w446]
                        frame No Error {
                          n252 = Send Notification(notification=w439, notifier=w440) -> ()  [unwired: 1 in, 2 out]
                        }
                        frame Error {
                          n253 = Unbundle(w446) -> ("tdms file out"=w445:refnum<k34>, "Tasks Out"=w444:refnum<k21>[], "DigitalTasks OUT"=w443:refnum<k21>[], "AnalogTaskOut"=w442:refnum<k21>[])  [unwired: 1 out]
                          n254 = local read "KillEvent"() -> (w450:refnum<user-event>[])
                          n255 = Bundle("tdms file out"=w445, "Tasks Out"=w444, "DigitalTasks OUT"=w443, "AnalogTaskOut"=w442) -> (w441:T23)  [unwired: 1 in]
                          n256 = call <vilib>:"Clear Errors.vi"("error in (no error)"=w447) -> ("error out"=w448:errorcluster)  [unwired: 6 in]
                          n257 = Index Array(array=w450) -> (element=w449:refnum<user-event>)  [unwired: 1 in]
                          n258 = Generate User Event(user event=w449, event data cluster=w441, error in=w448) -> ()  [unwired: 2 out]
                        }
                      }
                    }
                    frame Error {
                      n259 = property class="Bool (strict)"(reference=w453, "Value"=FALSE) -> ()  [unwired: 1 in, 2 out]
                      n260 = Unbundle By Name(w452) -> ("code"=w451:i32)
                      n261 = case shown="6" w451 {
                        tunnel: w452 -> [w455 _]
                        frame 0, Default {
                          n262 = call <vilib>:"Simple Error Handler.vi"("error in (no error)"=w455) -> ()  [unwired: 4 in, 5 out]
                        }
                        frame 6 {
                          n263 = call "overwrite error"() -> ()  [unwired: 10 in, 2 out]
                        }
                      }
                    }
                  }
                }
              }
            }
            event "Open Button", "Save Button": Value Change {
              n264 = event-data() -> ("CtlRef"=w457:refnum<vi>)  [unwired: 1 in, 4 out]
              n265 = control-ref of="Save Button"() -> (w459:refnum<vi>)
              n266 = control-ref of="Open Button"() -> (w460:refnum<vi>)
              n267 = Build Array(w460, w459) -> (w458:refnum<vi>[])
              n268 = Search 1D Array(1D array=w458, element=w457) -> (index of element=w456:i32)  [unwired: 1 in]
              n269 = case shown="1" w456 {
                frame 1 {
                  n270 = local read "XMLConfigControls"() -> (w461:refnum<vi>[])
                  n271 = control-ref of="This VI"() -> (w463:refnum<vi>)
                  n272 = call "storeControlXML.vi"("XMLoption"=XmlOption."Save Custom", "CallerVIref"=w463, "Control References"=w461) -> ()  [unwired: 2 in, 1 out]
                }
                frame 0, Default {
                  n273 = local read "XMLConfigControls"() -> (w464:refnum<vi>[])
                  n274 = control-ref of="This VI"() -> (w466:refnum<vi>)
                  n275 = call "storeControlXML.vi"("XMLoption"=XmlOption."Load Custom", "CallerVIref"=w466, "Control References"=w464) -> ()  [unwired: 2 in, 1 out]
                }
              }
            }
            event User Event {
              n276 = event-data() -> ("tdms file out"=w470:refnum<k34>, "Tasks Out"=w476:refnum<k21>[], "DigitalTasks OUT"=w475:refnum<k21>[], "AnalogOut"=w474:refnum<k21>[])  [unwired: 1 in, 3 out]
              n277 = Not A Number/Path/Refnum?(number/path/refnum=w470) -> (NaN/Path/Refnum?=w469:bool)
              n278 = case shown="False" w469 {
                tunnel: [w489 errorcluster {"status"=FALSE, "code"=0, "source"=""} ("error out")] -> w478
                tunnel: w470 -> [w485 _]
                frame False {
                  n279 = local read "Note"() -> (w484:string)
                  n280 = local read "TDMS Group Name"() -> (w483:string)
                  n281 = TDMS Set Properties(5:w484, 7:"Note" ("property names"), 10:w483, 11:w485) -> (0:w487:errorcluster, 3:w486:refnum<k34>)  [unwired: 2 in, 2 out]
                  n282 = TDMS Close(8:w487, 11:w486) -> (0:w488:errorcluster)  [unwired: 1 out]
                  n283 = call <vilib>:"Clear Errors.vi"("error in (no error)"=w488) -> ("error out"=w489:errorcluster)  [unwired: 6 in]
                }
                frame True {
                }
              }
              n284 = for {
                tunnel: w478 -> [w503]
                tunnel: [w502] -> w477
                tunnel: w476 -> [w501] mode=indexing
                n285 = call <vilib>:"DAQmx Clear Task.vi"("task in"=w501, "error in"=w503) -> ("error out"=w504:errorcluster)  [unwired: 13 in]
                n286 = call <vilib>:"Clear Errors.vi"("error in (no error)"=w504) -> ("error out"=w502:errorcluster)  [unwired: 6 in]
              }
              n287 = local read "DisableDuringRecord"() -> (w473:refnum<vi>[])
              n288 = local read "DisableDuringRun"() -> (w472:refnum<vi>[])
              n289 = for {
                tunnel: w477 -> [w499]
                tunnel: [w498] -> w480
                tunnel: w475 -> [w497] mode=indexing
                n290 = call <vilib>:"DAQmx Clear Task.vi"("task in"=w497, "error in"=w499) -> ("error out"=w500:errorcluster)  [unwired: 13 in]
                n291 = call <vilib>:"Clear Errors.vi"("error in (no error)"=w500) -> ("error out"=w498:errorcluster)  [unwired: 6 in]
              }
              n292 = Build Array (concatenate)(w472, w473) -> (w471:refnum<vi>[])
              n293 = for {
                tunnel: w480 -> [w495]
                tunnel: [w494] -> w481
                tunnel: w474 -> [w493] mode=indexing
                n294 = call <vilib>:"DAQmx Clear Task.vi"("task in"=w493, "error in"=w495) -> ("error out"=w496:errorcluster)  [unwired: 13 in]
                n295 = call <vilib>:"Clear Errors.vi"("error in (no error)"=w496) -> ("error out"=w494:errorcluster)  [unwired: 6 in]
              }
              n296 = for {
                tunnel: w471 -> [w492] mode=indexing
                n297 = property class="Ctl"(reference=w492, "DisabledEnum"=T15."Enabled" ("Disabled")) -> ()  [unwired: 1 in, 2 out]
              }
              n298 = property on="StartRecord" class="Bool (strict)"(error in=w481, "Value"=FALSE ("StartRecord")) -> (error out=w468:errorcluster)  [unwired: 1 in, 1 out]
              n299 = property on="Note" class="Str"(error in=w468, "Value"="") -> ()  [unwired: 1 in, 2 out]
            }
            event "Menu Ring": Value Change {
              n300 = event-data() -> ("NewVal"=w505:enum16{"Manual", "Column"})  [unwired: 1 in, 4 out]
              n301 = case shown="\"Manual\", Default" w505 {
                frame "Manual", Default {
                  w506 = T15."Disabled and Grayed Out" ("Disabled")
                  w507 = T15."Enabled" ("Disabled")
                  n302 = property on="Index" class="DigNum (strict)"("DisabledEnum"=w506) -> ()  [unwired: 2 in, 2 out]
                  n303 = property on="Up Button" class="Bool (strict)"("DisabledEnum"=w506) -> ()  [unwired: 2 in, 2 out]
                  n304 = property on="Down Button" class="Bool (strict)"("DisabledEnum"=w506) -> ()  [unwired: 2 in, 2 out]
                  n305 = property on="Last Index" class="DigNum (strict)"("DisabledEnum"=w507) -> ()  [unwired: 2 in, 2 out]
                  n306 = property on="First Index" class="DigNum (strict)"("DisabledEnum"=w507) -> ()  [unwired: 2 in, 2 out]
                }
                frame "Column" {
                  w508 = T15."Enabled" ("Disabled")
                  w510 = T15."Disabled" ("Disabled")
                  n307 = property on="Index" class="DigNum (strict)"("DisabledEnum"=w508) -> ()  [unwired: 2 in, 2 out]
                  n308 = property on="Up Button" class="Bool (strict)"("DisabledEnum"=w508) -> ()  [unwired: 2 in, 2 out]
                  n309 = property on="Down Button" class="Bool (strict)"("DisabledEnum"=w508) -> ()  [unwired: 2 in, 2 out]
                  n310 = local read "Index"() -> (w509:i32)
                  n311 = property on="Index" class="DigNum (strict)"("Val(Sgnl)"=w509) -> ()  [unwired: 2 in, 2 out]
                  n312 = property on="Last Index" class="DigNum (strict)"("DisabledEnum"=w510) -> ()  [unwired: 2 in, 2 out]
                  n313 = property on="First Index" class="DigNum (strict)"("DisabledEnum"=w510) -> ()  [unwired: 2 in, 2 out]
                }
              }
            }
            event "Index": Value Change {
              n314 = event-data() -> ("NewVal"=w511:i32)  [unwired: 1 in, 4 out]
              n315 = local read "HWSettings"() -> (w516:T5)
              n316 = Unbundle By Name(w516) -> ("Nr. of Rows"=w513:i32)
              n317 = Multiply(x=w513, y=w511) -> (x*y=w514:i32)
              n318 = Add(x=w514, y=w513) -> (x+y=w515:i32)
              n319 = Decrement(x=w515) -> (x-1=w512:i32)
              n320 = property on="Plot Properties" class="Clust (strict)"() -> ("Value"=w517:T25)  [unwired: 2 in, 2 out]
              n321 = Bundle By Name(cluster=w517, "First Index"=w514, "Last Index"=w512) -> (w518:T25)
              n322 = property on="Plot Properties" class="Clust (strict)"("Value"=w518) -> ()  [unwired: 2 in, 2 out]
            }
            event "Up Button", "Down Button": Value Change {
              n323 = event-data() -> ("CtlRef"=w520:refnum<vi>)  [unwired: 1 in, 4 out]
              n324 = control-ref of="Up Button"() -> (w526:refnum<vi>)
              n325 = control-ref of="Down Button"() -> (w525:refnum<vi>)
              n326 = property class="Bool (strict)"(reference=w520, "Value"=FALSE) -> ()  [unwired: 1 in, 2 out]
              n327 = Build Array(w525, w526) -> (w524:refnum<vi>[])
              n328 = local read "HWSettings"() -> (w521:T5)
              n329 = local read "Index"() -> (w522:i32)
              n330 = Search 1D Array(1D array=w524, element=w520) -> (index of element=w523:i32)  [unwired: 1 in]
              n331 = case shown="1" w523 {
                tunnel: w522 -> [w531 w537]
                tunnel: w521 -> [_ w536]
                frame 0, Default {
                  n332 = Decrement(x=w531) -> (x-1=w529:i32)
                  n333 = Less Or Equal To 0?(x=w529) -> (x <= 0?=w530:bool)
                  n334 = Select(t=0, s=w530, f=w529) -> (s? t:f=w527:i32)
                  n335 = property on="Index" class="DigNum (strict)"("Val(Sgnl)"=w527) -> ()  [unwired: 2 in, 2 out]
                }
                frame 1 {
                  n336 = Unbundle By Name(w536) -> ("Nr. of Columns"=w532:i32)
                  n337 = Increment(x=w537) -> (x+1=w533:i32)
                  n338 = Greater?(x=w533, y=w532) -> (0:w534:bool)
                  n339 = Select(t=w532, s=w534, f=w533) -> (s? t:f=w535:i32)
                  n340 = property on="Index" class="DigNum (strict)"("Val(Sgnl)"=w535) -> ()  [unwired: 2 in, 2 out]
                }
              }
            }
            event "Preview?": Value Change {
              n341 = event-data() -> ("NewVal"=w538:bool)  [unwired: 1 in, 4 out]
              n342 = case shown="False" w538 {
                frame False {
                  n343 = property on="TDMS file path" class="Path"("DisabledEnum"=T15."Enabled" ("Disabled")) -> ()  [unwired: 2 in, 2 out]
                  n344 = property on="StartRecord" class="Bool (strict)"("Strings [4]"=string[] ["START RECORDING", "STOP RECORDING"]) -> ()  [unwired: 2 in, 2 out]
                }
                frame True {
                  n345 = property on="TDMS file path" class="Path"("DisabledEnum"=T15."Disabled and Grayed Out" ("Disabled")) -> ()  [unwired: 2 in, 2 out]
                  n346 = property on="StartRecord" class="Bool (strict)"("Strings [4]"=string[] ["START PREVIEW", "STOP PREVIEW"]) -> ()  [unwired: 2 in, 2 out]
                }
              }
            }
            event Value Change {
              n347 = event-data() -> ("CtlRef"=w550:refnum<vi>, "OldVal"=w548:T6, "NewVal"=w549:T6)  [unwired: 1 in, 2 out]
              n348 = Array Size(array=w548) -> (size(s)=w552:i32)
              n349 = Array Size(array=w549) -> (size(s)=w551:i32)
              n350 = Less?(x=w552, y=w551) -> (x < y?=w545:bool)
              n351 = for {
                tunnel: w549 -> [w558] mode=indexing
                tunnel: w548 -> [w559] mode=indexing
                tunnel: [w553] -> w547 mode=indexing
                n352 = Unbundle(w558) -> ("AnalogOut (Volt)"=w556:dbl[])  [unwired: 1 out]
                n353 = Unbundle(w559) -> ("AnalogOut (Volt)"=w557:dbl[])  [unwired: 1 out]
                n354 = Array Size(array=w557) -> (size(s)=w554:i32)
                n355 = Array Size(array=w556) -> (size(s)=w555:i32)
                n356 = Less?(x=w554, y=w555) -> (x < y?=w553:bool)
              }
              n357 = Or Array Elements(Boolean array=w547) -> (logical OR=w544:bool)
              n358 = Or(x=w545, y=w544) -> (x .or. y?=w546:bool)
              n359 = case shown="False" w546 {
                tunnel: w550 -> [_ w568]
                tunnel: w549 -> [w562 _]
                tunnel: w548 -> [_ w567]
                frame False {
                  n360 = local read "AllTasks"() -> (w561:T1)
                  n361 = Unbundle By Name(w561) -> ("AnalogTaskOut"=w560:refnum<k21>[])
                  n362 = for {
                    tunnel: w562 -> [w566] mode=indexing
                    tunnel: w560 -> [w564] mode=indexing
                    n363 = Unbundle By Name(w566) -> ("AnalogOut (Volt)"=w565:dbl[])
                    n364 = call-poly <vilib>:"DAQmx Write.vi"("task/channels in"=w564, "data"=w565) -> ("error out"=w563:errorcluster)  [unwired: 11 in, 2 out]
                    n365 = call <vilib>:"Clear Errors.vi"("error in (no error)"=w563) -> ()  [unwired: 6 in, 1 out]
                  }
                }
                frame True {
                  n366 = property class="Arr (strict)"(reference=w568, "Value"=w567) -> ()  [unwired: 1 in, 2 out]
                  n367 = call "Display Message to User3"() -> ()  [unwired: 10 in, 2 out]
                }
              }
            }
          }
        }
      }
      frame "Close" {
        n368 = flat-sequence {
          frame #0 {
            n369 = local read "XMLConfigControls"() -> (w571:refnum<vi>[])
            n370 = local read "KillEvent"() -> (w574:refnum<user-event>[])
            n371 = control-ref of="This VI"() -> (w573:refnum<vi>)
            n372 = for {
              tunnel: w574 -> [w575] mode=indexing
              n373 = Destroy User Event(user event=w575) -> ()  [unwired: 1 in, 1 out]
            }
            n374 = call "storeControlXML.vi"("XMLoption"=XmlOption."Save Default", "CallerVIref"=w573, "Control References"=w571) -> ()  [unwired: 2 in, 1 out]
          }
          frame #1 {
            n375 = control-ref of="This VI"() -> (w576:refnum<vi>)
            n376 = invoke class="VI" method="FP.Close"(reference=w576) -> ()  [unwired: 2 in, 3 out]
          }
        }
      }
      frame "Init2" {
        n377 = flat-sequence {
          frame #0 {
            n378 = control-ref of="AutoNr"() -> (w620:refnum<vi>)
            n379 = control-ref of="Preview?"() -> (w621:refnum<vi>)
            n380 = control-ref of="OverWrite?"() -> (w622:refnum<vi>)
            n381 = control-ref of="HWSettings"() -> (w615:refnum<vi>)
            n382 = control-ref of="AnalogSettings"() -> (w612:refnum<vi>)
            n383 = control-ref of="LUT"() -> (w613:refnum<vi>)
            n384 = control-ref of="Digital Out Tasks"() -> (w617:refnum<vi>)
            n385 = control-ref of="AnalogInSettings"() -> (w618:refnum<vi>)
            n386 = control-ref of="RowConfigFile"() -> (w616:refnum<vi>)
            n387 = control-ref of="TDMS file path"() -> (w619:refnum<vi>)
            n388 = Build Array(w619, w620, w621, w622, w618, w617, w616, w615) -> (w614:refnum<vi>[])
            "DisableDuringRun" <- w614
            n389 = Build Array(w613, w612) -> (→"DisableDuringRecord":refnum<vi>[])
            n390 = for {
              tunnel: w614 -> [w624] mode=indexing
              n391 = property class="Ctl"(reference=w624, "DisabledEnum"=T15."Enabled" ("Disabled")) -> ()  [unwired: 1 in, 2 out]
            }
          }
        }
        n392 = local write "TDMS file path"(path "C:/Users/DAQ/Desktop/test_001.tdms" ("TDMS file path")) -> ()
        n393 = local write "TDMS Group Name"("MultiplexRecord" ("TDMS Group Name")) -> ()
        n394 = control-ref of="BitSwitch"() -> (w581:refnum<vi>)
        n395 = control-ref of="Counter Setup"() -> (w584:refnum<vi>)
        n396 = control-ref of="Sample Clock Export"() -> (w585:refnum<vi>)
        n397 = control-ref of="HWSettings"() -> (w590:refnum<vi>)
        n398 = control-ref of="Referece Clock Setup"() -> (w580:refnum<vi>)
        n399 = control-ref of="AnalogInSettings"() -> (w577:refnum<vi>)
        n400 = control-ref of="Digital Out Tasks"() -> (w587:refnum<vi>)
        n401 = control-ref of="AnalogSettings"() -> (w588:refnum<vi>)
        n402 = control-ref of="LUT"() -> (w589:refnum<vi>)
        n403 = control-ref of="RowConfigFile"() -> (w586:refnum<vi>)
        n404 = Build Array(w577, w580, w584, w585, w586, w587, w588, w589, w590, w581) -> (w579:refnum<vi>[])
        "XMLConfigControls" <- w579
        n405 = control-ref of="This VI"() -> (w583:refnum<vi>)
        n406 = call "storeControlXML.vi"("XMLoption"=XmlOption."Load Default", "CallerVIref"=w583, "Control References"=w579) -> ("Error Out"=w578:errorcluster)  [unwired: 2 in]
        n407 = case shown="Error" w578 {
          frame No Error {
          }
          frame Error {
            n408 = property class="DAQmx System"() -> (error out=w598:errorcluster, "DevNames"=w599:tag[])  [unwired: 2 in, 1 out]
            n409 = for {
              tunnel: w599 -> [w605] mode=indexing
              shift-right: [w603] -> w596
              shift-left: w598 -> [w610]
              shift-right: [w607] -> w597
              shift-left: T6 [] ("AnalogSettings") -> [w608]
              i -> [w609]
              n410 = property class="DAQmx Device"(error in=w610, "Active Device"=w605) -> (error out=w603:errorcluster, "AO.PhysicalChans"=w606:tag[])  [unwired: 1 in, 1 out]
              n411 = Array Size(array=w606) -> (size(s)=w601:i32)
              n412 = Initialize Array(0.0 ("element"), w601) -> (w602:dbl[])
              n413 = Bundle(w602, w605) -> (w604:cluster{dbl[], tag})  [unwired: 1 in]
              n414 = Insert Into Array(array=w608, index=w609, new element=w604) -> (w607:T6)
            }
            n415 = call <vilib>:"General Error Handler.vi"("error in (no error)"=w596) -> ()  [unwired: 10 in, 5 out]
            n416 = local write "AnalogSettings"(w597) -> ()
          }
        }
      }
    }
  }
